vi "FaulhaberV3.vi"(5 "Sub":u8 format="%02x", 6 "Knoten":u8=1, 7 "Index":u16=24640 format="%04x", 10 "SendValue":u8[](array[numeric])=[0, 0] format="%02x", 11 "Befehl":T1(ring)=enum."SDORead") -> (3 "Send":u8[](array[numeric])=[83, 9, 1, 1, 64, 96, 0, 0, 0, 131, 69] format="%02x")   [LabVIEW 2011]
panel:
  # "er gibt immer antwort!"
  # "53,9,1,2,40,60,00,06,00,2C,45\nS,Length,Node,SDOWrite,Adr6040.00 Data00 60, CRC, Eof \"E\""
  # "6040.00=6 switch On"
  # "CRC.Polynon D5 byte2-N (Ohne S)"
  # "1000-1FFF Communikation\n2000-5FFF hersteller\n6000-9FFF StandadGerät"
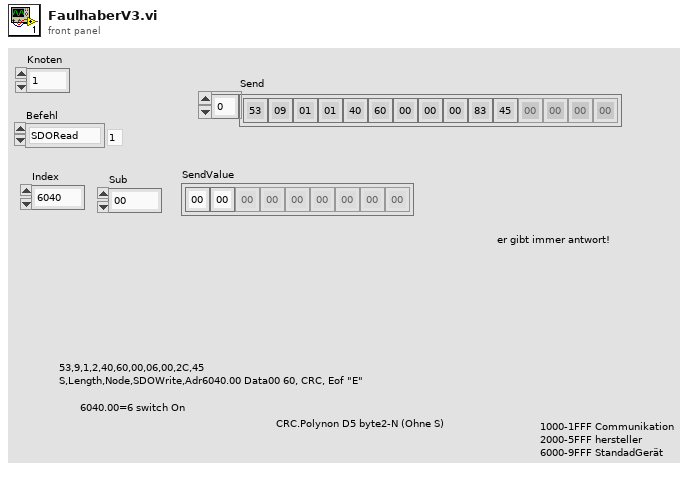
[diagram p1: front panel]
types:
  T1 = enum8{"Bootup", "SDORead", "SDOWrite", "SDOErrror", "Controlword", "Statusword", "TraceLog", "Emcy", "SDOBlockReadInit", "SDOBlockReadUpload", "SDOBlockReadEnd", "SDOBlockWriteInit", "SDOBlockWriteDownload", "SDOBlockWriteEnd"}
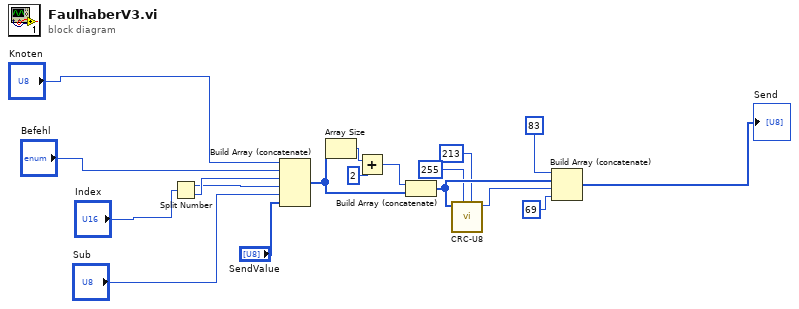
[diagram p0: block diagram]
diagram:
  n1 = Split Number(x="Index") -> (hi(x)=w14:u8, lo(x)=w15:u8)
  n2 = Build Array (concatenate)("Knoten", "Befehl", w15, w14, "Sub", "SendValue") -> (w9:u8[])
  n3 = Array Size(array=w9) -> (size(s)=w12:i32)
  n4 = Add(x=w12, y=2) -> (x+y=w7:i32)
  n5 = Build Array (concatenate)(w7, w9) -> (w6:i32[])
  n6 = call "CRC-U8.vi"("Polynom"=u8 213, "Start"=u8 255, "Send"=w6) -> ("CRC"=w5:u8)  [unwired: 8 in]
  n7 = Build Array (concatenate)(83, w6, w5, u8 69) -> (→"Send":i32[])
